vi "Main.vi"() -> ()   [LabVIEW 2020]
panel:
  in  "vi path change":path
  in  "vi path":path=path "C:/Users/Kamil/Documents/LabView_Project/Home.vi"
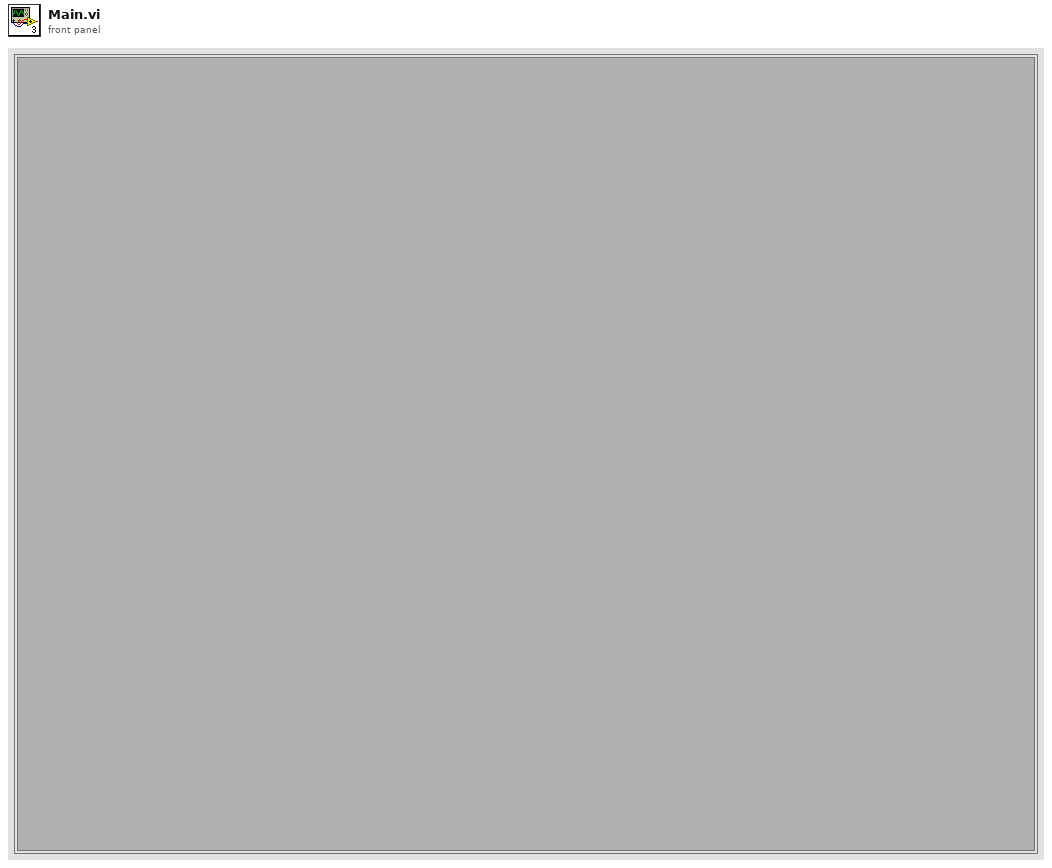
[diagram p1: front panel]
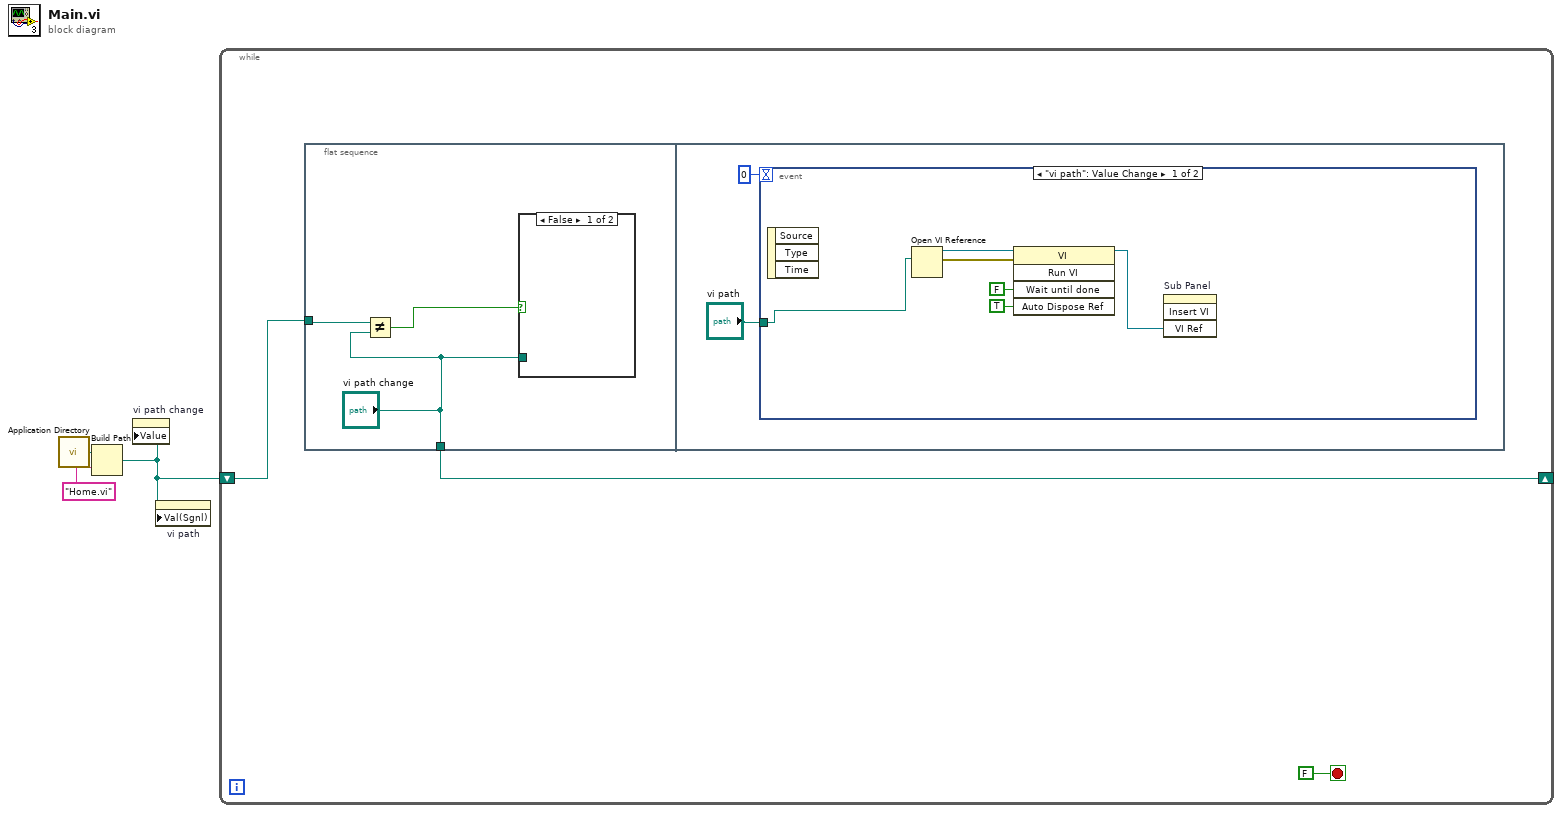
[diagram p0: block diagram]
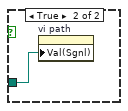
[diagram p2: hidden frame]
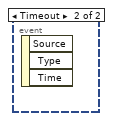
[diagram p3: hidden frame]
diagram:
  n1 = call <vilib>:"Application Directory.vi"() -> ("Application Directory"=w2:path)
  n2 = Build Path(base path=w2, name or relative path="Home.vi") -> (appended path=w1:path)
  n3 = property on="vi path change" class="Path"("Value"=w1) -> ()  [unwired: 2 in, 2 out]
  n4 = property on="vi path" class="Path"("Val(Sgnl)"=w1) -> ()  [unwired: 2 in, 2 out]
  n5 = while {
    shift-right: [w5] -> _
    shift-left: w1 -> [w4]
    stop <- FALSE stop-if-true
    n6 = flat-sequence {
      tunnel: ["vi path change"] -> w5
      tunnel: w4 -> [w9]
      frame #0 {
        n7 = Not Equal?(x=w9, y="vi path change") -> (x != y?=w7:bool)
        n8 = case shown="False" w7 {
          tunnel: "vi path change" -> [_ w10]
          frame False {
          }
          frame True {
            n9 = property on="vi path" class="Path"("Val(Sgnl)"=w10) -> ()  [unwired: 2 in, 2 out]
          }
        }
      }
      frame #1 {
        n10 = event shown="[0] \"vi path\": Value Change" {
          selector: _ -> [_ _]
          dyn-events: _ -> [_ _]
          timeout: 0 -> [_ _]
          tunnel: "vi path" -> [w16 _]
          event "vi path": Value Change {
            n11 = event-data() -> ()  [unwired: 1 in, 3 out]
            n12 = Open VI Reference(vi path=w16) -> (vi reference=w18:refnum<vi>, error out=w17:errorcluster)  [unwired: 5 in]
            n13 = invoke class="VI" method="Run VI"(reference=w18, error in=w17, "Wait until done"=FALSE ("Wait Until Done"), "Auto Dispose Ref"=TRUE ("Auto Dispose Reference")) -> (reference out=w14:refnum<vi>)  [unwired: 1 in, 4 out]
            n14 = invoke on="Sub Panel" class="SubPnl" method="Insert VI"("VI Ref"=w14) -> ()  [unwired: 3 in, 4 out]
          }
          event Timeout {
            n15 = event-data() -> ()  [unwired: 1 in, 3 out]
          }
        }
      }
    }
  }
